vi "Create Convolution 32f.vi"(8 "Error In":errorcluster, 9 "Convolution Dimensions":T4={"Depth"=1, "Height"=1, "Width"=1} {"Width" min=1; "Height" min=1; "Depth" min=1}, 10 "Memory Object":T1 {"Dimension"."Width" min=1; "Dimension"."Height" min=1; "Dimension"."Depth" min=1}, 11 "Device In":T2) -> (0 "Error Out":errorcluster, 3 "Convolution Object":T6 {"Convolved Memory Object"."Dimension"."Width" min=1; "Convolved Memory Object"."Dimension"."Height" min=1; "Convolved Memory Object"."Dimension"."Depth" min=1; "Kernel Memory Object"."Dimension"."Width" min=1; "Kernel Memory Object"."Dimension"."Height" min=1; "Kernel Memory Object"."Dimension"."Depth" min=1})   [LabVIEW 2012, in "OpenCLV x64.lvlib"]
doc: "Create a Convolution Object based on the input dimensions. The convolution can be either 2D or 3D, depending on the combination of the kernel and the dataset."
uses:
  OpenCLV x64.lvlib
  Controls/Device ID.ctl
  Controls/Convolution Object.ctl
  Controls/Program Handle.ctl
  Controls/Memory Object.ctl
  Controls/Memory ID.ctl
  User Controls/Array Dimensions.ctl
  Controls/Memory Type.ctl
  Allocate Memory/AllocateMemory_32f.vi
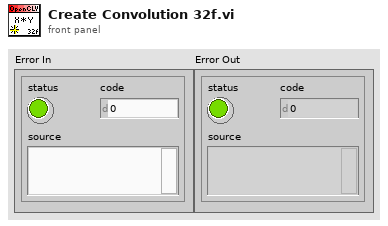
[diagram p1: front panel]
types:
  T1 = typedef "OpenCLV x64.lvlib/Memory Object.ctl" = cluster{"Device ID":T2, "Memeroy ID":T3, "Dimension":T4, "Memory Type":T5}
  T2 = typedef "OpenCLV x64.lvlib/Device ID.ctl" = u64
  T3 = typedef "OpenCLV x64.lvlib/Memory ID.ctl" = u64
  T4 = typedef "Array Dimensions.ctl" = cluster{"Depth":u64, "Height":u64, "Width":u64}
  T5 = typedef "OpenCLV x64.lvlib/Memory Type.ctl" = enum16{"32f", "u8", "i8", "u16", "i16", "u32", "i32", "64f"}
  T6 = typedef "OpenCLV x64.lvlib/Convolution Object.ctl" = cluster{"Device In":T2, "Program Handle":T7, "Kernel Memory Object":T1, "Convolved Memory Object":T1}
  T7 = typedef "OpenCLV x64.lvlib/Program Handle.ctl" = u64
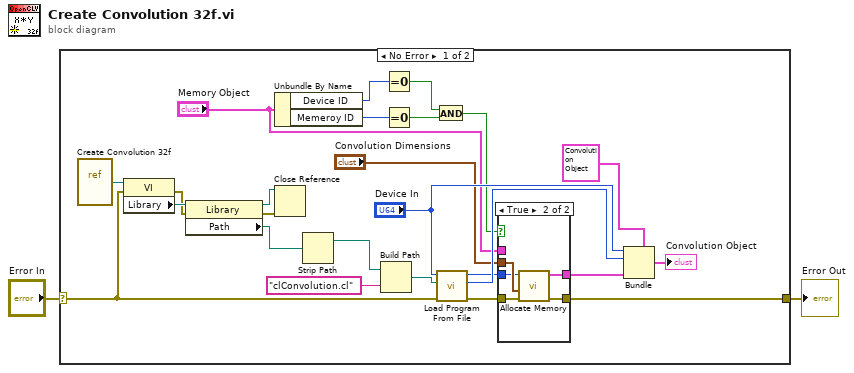
[diagram p0: block diagram]
diagram:
  n1 = case shown="No Error" "Error In" {
    selector: "Error In" -> [w3 w35]
    tunnel: [w14 w35] -> w1
    frame No Error {
      n2 = vi-ref "Create Convolution 32f.vi"() -> (w23:refnum<vi>)
      n3 = property class="VI"(reference=w23, error in=w3) -> (error out=w4:errorcluster, "Library"=w25:refnum<vi>)  [unwired: 1 out]
      n4 = property class="Library"(reference=w25, error in=w4) -> (reference out=w5:refnum<vi>, error out=w6:errorcluster, "Path"=w24:path)
      n5 = Unbundle By Name("Memory Object") -> ("Device ID"=w11:T2, "Memeroy ID"=w10:T3)
      n6 = Close Reference(reference=w5, error in (no error)=w6) -> ()  [unwired: 1 out]
      n7 = Strip Path(path=w24) -> (stripped path=w27:path)  [unwired: 1 out]
      n8 = Build Path(base path=w27, name or relative path="clConvolution.cl") -> (appended path=w22:path)
      n9 = Equal To 0?(x=w11) -> (x = 0?=w9:bool)
      n10 = Equal To 0?(x=w10) -> (x = 0?=w12:bool)
      n11 = And(x=w9, y=w12) -> (x .and. y?=w8:bool)
      n12 = call "Load Program From File.vi"("Error In"=w3, "Program Path"=w22, "Device In"="Device In") -> ("Error Out"=w17:errorcluster, "Program Handle"=w21:T7, "Device Out"=w16:T2)  [unwired: 6 in]
      n13 = case shown="True" w8 {
        tunnel: "Convolution Dimensions" -> [_ w34]
        tunnel: w17 -> [w29 w33]
        tunnel: [w28 w32] -> w15
        tunnel: [w29 w31] -> w14
        tunnel: w16 -> [_ w30]
        tunnel: "Memory Object" -> [w28 _]
        frame False {
        }
        frame True {
          n14 = call-poly "Allocate Memory.vi"("Error In"=w33, "Dimension"=w34, "Device In"=w30) -> ("Error Out"=w31:errorcluster, "Memory Object"=w32:T1)  [unwired: 6 in, 1 out]
        }
      }
      n15 = Bundle(cluster=T6 {"Device In"=0, "Program Handle"=0, "Kernel Memory Object"={"Device ID"=0, "Memeroy ID"=0, "Dimension"={"Depth"=0, "Height"=0, "Width"=0}, "Memory Type"=enum."32f"}, "Convolved Memory Object"={"Device ID"=0, "Memeroy ID"=0, "Dimension"={"Depth"=0, "Height"=0, "Width"=0}, "Memory Type"=enum."32f"}} ("Convolution Object 2"), "Device In"="Device In", "Program Handle"=w21, "Convolved Memory Object"=w15) -> (→"Convolution Object":T6)  [unwired: 1 in]
    }
    frame Error {
    }
  }
  "Error Out" <- w1
